vi "RD_WR init.vi"(8 "error in":errorcluster, 10 "N_moduls":i32) -> (0 "error":errorcluster, 3 "RD_WR param":T1)   [LabVIEW 2019, in "ICPCON_Param.lvlib"]
uses:
  ICPCON_Param.lvlib
  ICPCON Param.ctl
  Eth timeouts.ctl
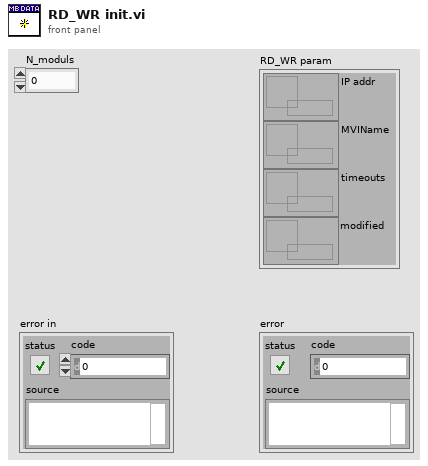
[diagram p1: front panel]
types:
  T1 = typedef "ICPCON_Param.lvlib/ICPCON Param.ctl" = cluster{"IP addr":refnum<data-value>, "MVIName":refnum<data-value>, "timeouts":refnum<data-value>, "modified":refnum<data-value>}
  T2 = cluster{"Remote IP Address":string, "Remote Port":u16}
  T3 = typedef "ICPCON_Param.lvlib/Eth timeouts.ctl" = cluster{"conn_timeout":i32, "reconn_timeout":i32, "N attempt max":i32, "t_reset_TTL":i32, "write_timeout":i32, "read_timeout":i32, "period":i32}
  T4 = cluster{"Remote IP Address":string, "Remote Port":u16}[]
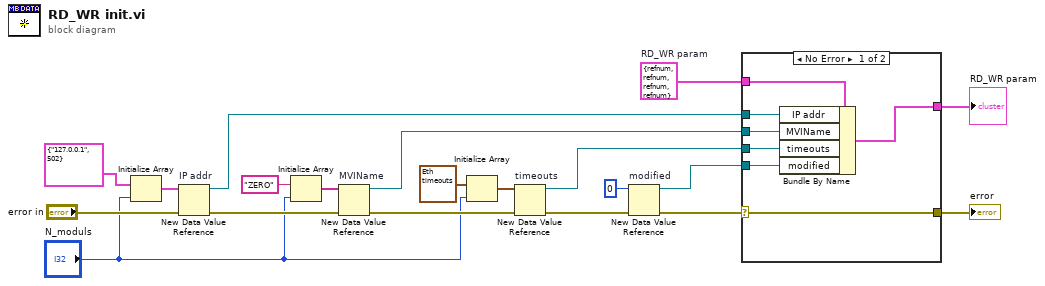
[diagram p0: block diagram]
diagram:
  w7 = T1 {"IP addr"=refnum, "MVIName"=refnum, "timeouts"=refnum, "modified"=refnum}  # RD_WR param
  n1 = Initialize Array(T2 {"Remote IP Address"="127.0.0.1", "Remote Port"=502} ("IP address"), "N_moduls") -> (w18:T4)
  n2 = New Data Value Reference "IP addr"(data value=w18, error in="error in") -> (data value reference=w13:refnum<data-value>, error out=w11:errorcluster)
  n3 = Initialize Array("ZERO" ("MVIName"), "N_moduls") -> (w19:string[])
  n4 = New Data Value Reference "MVIName"(data value=w19, error in=w11) -> (data value reference=w17:refnum<data-value>, error out=w12:errorcluster)
  n5 = Initialize Array(T3 {"conn_timeout"=1000, "reconn_timeout"=3000, "N attempt max"=3, "t_reset_TTL"=120000, "write_timeout"=50, "read_timeout"=500, "period"=100} ("timeouts"), "N_moduls") -> (w20:T3[])
  n6 = New Data Value Reference "timeouts"(data value=w20, error in=w12) -> (data value reference=w16:refnum<data-value>, error out=w4:errorcluster)
  n7 = New Data Value Reference "modified"(data value=u8 0 ("modified"), error in=w4) -> (data value reference=w1:refnum<data-value>, error out=w3:errorcluster)
  n8 = case shown="No Error" w3 {
    selector: w3 -> [w22 w29]
    tunnel: w13 -> [w26 _]
    tunnel: w17 -> [w25 _]
    tunnel: [w22 w29] -> w5
    tunnel: w16 -> [w24 _]
    tunnel: w7 -> [w27 w28]
    tunnel: [w23 w28] -> w6
    tunnel: w1 -> [w21 _]
    frame No Error {
      n9 = Bundle By Name(cluster=w27, "IP addr"=w26, "MVIName"=w25, "timeouts"=w24, "modified"=w21) -> (w23:T1)
    }
    frame Error {
    }
  }
  "error" <- w5
  "RD_WR param" <- w6
